vi "Gen Voltage Update.vi"() -> ()   [LabVIEW 2010]
doc: "I. Description:\nThis example demonstrates how to output a single Voltage Update (Sample) to an Analog Output Channel.\n\nII. Instructions for Running:\n1. Select the Physical Channel to correspond to where your signal is output on the DAQ device.\n2. Enter the Minimum and Maximum Voltage Ranges\nNote: Use the Acq One Sample example to verify you are generating the correct output on the DAQ device\n\nIII. Block Diagram Steps:\n1. Create an Analog Output Voltage Channel\n2. Use the Write VI to Output 1 Sample to 1 Channel on the Data\nAcquisition Card. \n3. Call the Clear Task VI to clear the Task.\n4. Use the popup dialog box to display an error if any. \n\nIV. I/O Connections Overview:\nMake sure your signal output terminal matches the Physical Channel I/O Control. For further connection information, refer to your hardware reference manual."
uses:
  <vilib>/Utility/error.llb/DialogType.ctl
  <vilib>/DAQmx/write.llb/DAQmx Write (Analog DBL 1Chan 1Samp).vi
  <vilib>/DAQmx/create/channels.llb/DAQmx Create Channel (AO-Voltage-Basic).vi
  <vilib>/daqmx/miscellaneous.llb/DAQmx Fill In Error Info.vi
panel:
  in  "Voltage Output":dbl(slide)=1.0 scale=-10.0..9.995 scale format="%.3f"
  in  "Maximum Value":dbl=10.0 format="%0.2f"
  in  "Minimum Value":dbl=-10.0 format="%0.2f"
  in  "Physical Channel":tag="Dev1/ao0"
  # "For instructions, select Help>>Show Context Help"
  # "Channel Parameters"
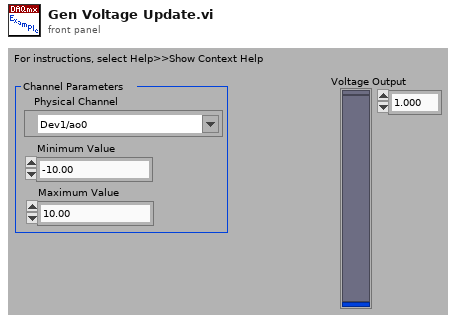
[diagram p1: front panel]
types:
  T1 = typedef "DialogType.ctl" = u16
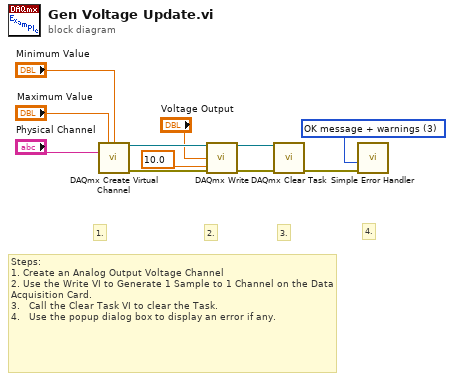
[diagram p0: block diagram]
diagram:
  w4 = T1 3 items=["no dialog", "OK message", "continue or stop message", "OK message + warnings", "continue/stop + warnings"] ("type of dialog (OK msg:1)")
  # "4."
  # "2."
  # "Steps: \n1. Create an Analog Output Voltage Channel\n2. Use the Write VI to Generate 1 Sample to 1 Channel on the Data Acquisition Card.  \n3.   Call the Clear Task VI to clear the Task.\n4.   Use the popup dialog box to display an error if any."
  # "3."
  # "1."
  n1 = call-poly <vilib>:"DAQmx Create Virtual Channel.vi"("maximum value"="Maximum Value", "minimum value"="Minimum Value", "physical channels"="Physical Channel") -> ("task out"=w7:refnum<k21>, "error out"=w8:errorcluster)  [unwired: 11 in]
  n2 = call-poly <vilib>:"DAQmx Write.vi"("task/channels in"=w7, "data"="Voltage Output", "timeout"=10.0, "error in"=w8) -> ("task out"=w2:refnum<k21>, "error out"=w3:errorcluster)  [unwired: 9 in, 1 out]
  n3 = call <vilib>:"DAQmx Clear Task.vi"("task in"=w2, "error in"=w3) -> ("error out"=w1:errorcluster)  [unwired: 13 in]
  n4 = call <vilib>:"Simple Error Handler.vi"("type of dialog (OK msg:1)"=w4, "error in (no error)"=w1) -> ()  [unwired: 3 in, 5 out]
